vi "De-Nan.vi"(11 "output in":dbl) -> (3 "output out":dbl)   [LabVIEW 2013]
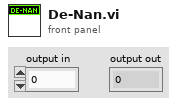
[diagram p1: front panel]
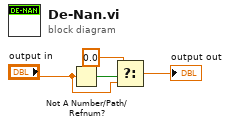
[diagram p0: block diagram]
diagram:
  n1 = Not A Number/Path/Refnum?(number/path/refnum="output in") -> (NaN/Path/Refnum?=w1:bool)
  n2 = Select(t=0.0, s=w1, f="output in") -> (s? t:f=→"output out":dbl)
